vi "Fill FN - Active (SubVI).vi"(0 "Signals IN":T2={"Dispense"=FALSE, "Fill"=FALSE, "Spray"=FALSE, "Drain"=TRUE, "Complete"=FALSE, "Fill Error"=FALSE, "Disp. Error"=FALSE, "Fill Timeout"=FALSE, "Disp. Timeout"=FALSE, "Purge"=TRUE}, 1 "Values IN":T3 {"Drain Time (s)" format="%.2f"; "Drain Rate (g/sec)" format="%.2f"}, 2 "Measured Mass (g)":dbl(knob) scale=0.0..1000.0, 3 "Settings":T1={"ON Settings"={"Enable Dynamic Setpoint?"=TRUE, "Enable Dynamic Dispense Time?"=TRUE, "Enable Drain Rate Functions"=TRUE, "Dispense Sample Time (s)"=0.1, "Mass Average Samples"=20, "ON Timeout (sec)"=300.0, "1st Setpoint (% of Target)"=90.0, "2nd Setpoint (% of Target)"=95.0, "3rd Setpoint (% of Target)"=100.0, "Measure Dispense Delay (sec)"=10.0, "Minimum Spray Time (s)"=2.0, "Pump Reverse Time (s)"=10.0}, "OFF Settings"={"Drain Sample Time (s)"=0.1, "Drain Rate Ave Size"=100, "Drain Rate Limits (± g/sec)"=100.0, "Level Slope Range (± g/sec)"=0.05, "OFF Timeout (sec)"=300.0, "Near SP Slope Level (± g/sec)"=0.005, "Near Setpoint Threshold (%)"=99.0}, "Overshoot Settings"={"Time Limit (s)"=30.0, "Container MAX (g)"=1500.0, "Max FILL Slope (+/- g/sec)"=100.0, "% Overshot to Enable (>)"=3.0}, "FILL Timeout (s)"=300.0, "Full \nSettle Time (s)"=30.0, "Pre-Hydrate \nSpray Time (s)"=0.0, "Pre-Hydrate \nWait Time (s)"=10.0, "m Value "=1.0, "b Value"=0.0, "Enable Overshoot Adjust?"=FALSE} {"ON Settings"."Pump Reverse Time (s)" min=0.0 max=60.0; "OFF Settings"."Near SP Slope Level (± g/sec)" format="%.3g"; "OFF Settings"."Level Slope Range (± g/sec)" format="%.3g"}, 5 "Fill Case Change?":bool, 7 "Initial Mass (g)":dbl, 9 "FILL Setpoint (g)":dbl) -> (14 "Signals OUT":T2={"Dispense"=FALSE, "Fill"=FALSE, "Spray"=FALSE, "Drain"=TRUE, "Complete"=FALSE, "Fill Error"=FALSE, "Disp. Error"=FALSE, "Fill Timeout"=FALSE, "Disp. Timeout"=FALSE, "Purge"=TRUE}, 15 "Values OUT":T3, 17 "Fill Timeout":bool, 19 "Case Complete":bool)   [LabVIEW 2011]
panel:
  # "ONLY ADJUST\nBOLD VALUES!"
  # "Corrected Mass = SDC Mass * m + b"
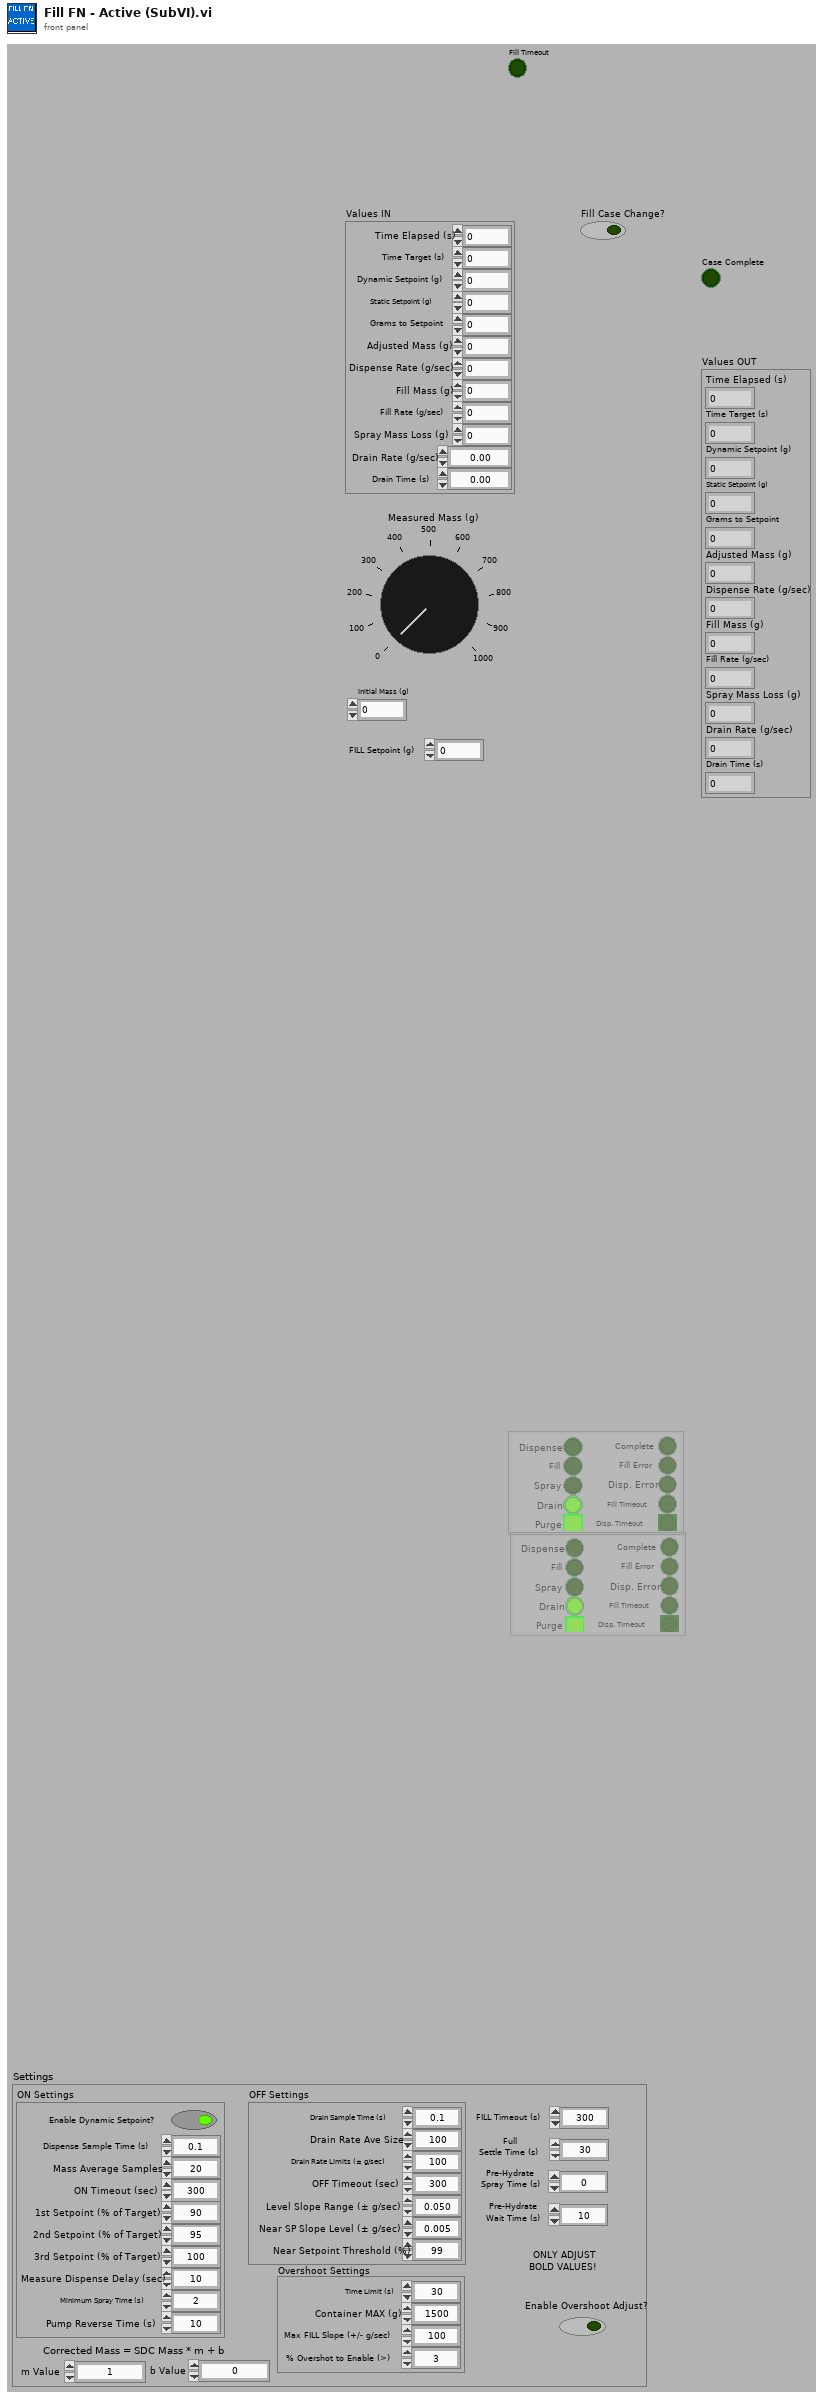
[diagram p1: front panel]
types:
  T1 = cluster{"ON Settings":cluster{"Enable Dynamic Setpoint?":bool, "Enable Dynamic Dispense Time?":bool, "Enable Drain Rate Functions":bool, "Dispense Sample Time (s)":dbl, "Mass Average Samples":i32, "ON Timeout (sec)":dbl, "1st Setpoint (% of Target)":dbl, "2nd Setpoint (% of Target)":dbl, "3rd Setpoint (% of Target)":dbl, "Measure Dispense Delay (sec)":dbl, "Minimum Spray Time (s)":dbl, "Pump Reverse Time (s)":dbl}, "OFF Settings":cluster{"Drain Sample Time (s)":dbl, "Drain Rate Ave Size":i32, "Drain Rate Limits (± g/sec)":dbl, "Level Slope Range (± g/sec)":dbl, "OFF Timeout (sec)":dbl, "Near SP Slope Level (± g/sec)":dbl, "Near Setpoint Threshold (%)":dbl}, "Overshoot Settings":cluster{"Time Limit (s)":dbl, "Container MAX (g)":dbl, "Max FILL Slope (+/- g/sec)":dbl, "% Overshot to Enable (>)":dbl}, "FILL Timeout (s)":dbl, "Full \nSettle Time (s)":dbl, "Pre-Hydrate \nSpray Time (s)":dbl, "Pre-Hydrate \nWait Time (s)":dbl, "m Value ":dbl, "b Value":dbl, "Enable Overshoot Adjust?":bool}
  T2 = cluster{"Dispense":bool, "Fill":bool, "Spray":bool, "Drain":bool, "Complete":bool, "Fill Error":bool, "Disp. Error":bool, "Fill Timeout":bool, "Disp. Timeout":bool, "Purge":bool}
  T3 = cluster{"Time Elapsed (s)":dbl, "Time Target (s)":dbl, "Dynamic Setpoint (g)":dbl, "Static Setpoint (g)":dbl, "Grams to Setpoint":dbl, "Adjusted Mass (g)":dbl, "Dispense Rate (g/sec)":dbl, "Fill Mass (g)":dbl, "Fill Rate (g/sec)":dbl, "Spray Mass Loss (g)":dbl, "Drain Rate (g/sec)":dbl, "Drain Time (s)":dbl}
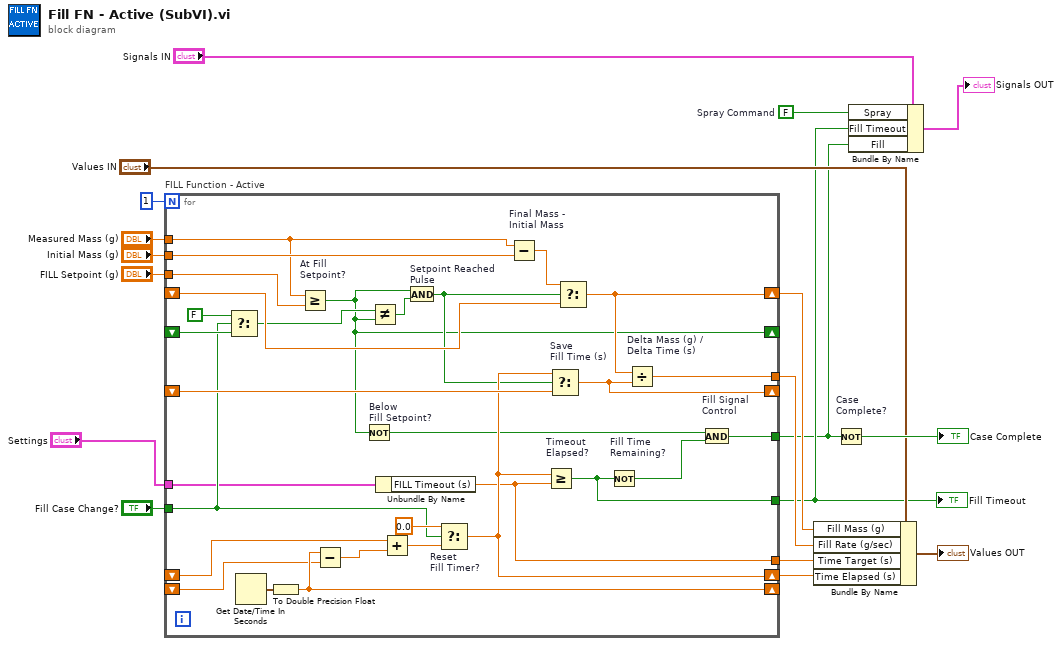
[diagram p0: block diagram]
diagram:
  w4 = FALSE  # Spray Command
  n1 = for "FILL Function - Active" {
    N: 1 -> [_]
    shift-right: [w38] -> w13
    shift-left: _ -> [w48]
    shift-right: [w45] -> _
    shift-left: _ -> [w44]
    tunnel: "Measured Mass (g)" -> [w28]
    tunnel: "FILL Setpoint (g)" -> [w43]
    tunnel: "Fill Case Change?" -> [w26]
    shift-right: [w24] -> _
    shift-left: _ -> [w32]
    shift-right: [w35] -> _
    shift-left: _ -> [w39]
    tunnel: "Initial Mass (g)" -> [w37]
    tunnel: [w36] -> w16
    shift-right: [w30] -> w15
    shift-left: _ -> [w34]
    tunnel: "Settings" -> [w25]
    tunnel: [w21] -> w5
    tunnel: [w20] -> w6
    tunnel: [w19] -> w14
    n2 = Select(t=FALSE ("y"), s=w26, f=w32) -> (s? t:f=w31:bool)
    n3 = Get Date/Time In Seconds() -> (seconds since 1Jan1904=w47:timestamp)
    n4 = To Double Precision Float(number=w47) -> (double precision float=w45:dbl)
    n5 = Greater Or Equal? "At Fill\nSetpoint?"(x=w28, y=w43) -> (x >= y?=w24:bool)
    n6 = Subtract(x=w45, y=w44) -> (x-y=w41:dbl)
    n7 = Not "Below\nFill Setpoint?"(x=w24) -> (.not. x?=w23:bool)
    n8 = Not Equal?(x=w31, y=w24) -> (x != y?=w42:bool)
    n9 = Unbundle By Name(w25) -> ("FILL Timeout (s)"=w19:dbl)
    n10 = Add(x=w48, y=w41) -> (x+y=w46:dbl)
    n11 = And "Setpoint Reached\nPulse"(x=w24, y=w42) -> (x .and. y?=w29:bool)
    n12 = Select "Reset\nFill Timer?"(t=0.0, s=w26, f=w46) -> (s? t:f=w38:dbl)
    n13 = Subtract "Final Mass -\nInitial Mass"(x=w28, y=w37) -> (x-y=w27:dbl)
    n14 = Greater Or Equal? "Timeout\nElapsed?"(x=w38, y=w19) -> (x >= y?=w20:bool)
    n15 = Select "Save\nFill Time (s)"(t=w38, s=w29, f=w39) -> (s? t:f=w35:dbl)
    n16 = Select(t=w27, s=w29, f=w34) -> (s? t:f=w30:dbl)
    n17 = Not "Fill Time\nRemaining?"(x=w20) -> (.not. x?=w22:bool)
    n18 = Divide "Delta Mass (g) /\nDelta Time (s)"(x=w30, y=w35) -> (x/y=w36:dbl)
    n19 = And "Fill Signal\nControl"(x=w23, y=w22) -> (x .and. y?=w21:bool)
  }
  "Fill Timeout" <- w6
  n20 = Bundle By Name(cluster="Values IN", "Fill Mass (g)"=w15, "Fill Rate (g/sec)"=w16, "Time Target (s)"=w14, "Time Elapsed (s)"=w13) -> (→"Values OUT":T3)
  n21 = Not "Case\nComplete?"(x=w5) -> (.not. x?=→"Case Complete":bool)
  n22 = Bundle By Name(cluster="Signals IN", "Spray"=w4, "Fill Timeout"=w6, "Fill"=w5) -> (→"Signals OUT":T2)
